vi "counter_polling.vi"() -> ()   [LabVIEW 2018]
panel:
  in  "Button":bool
  in  "stop":bool
  out "Count":u32
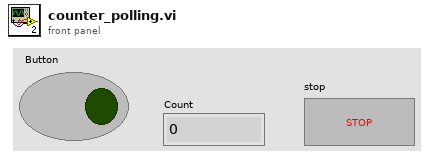
[diagram p1: front panel]
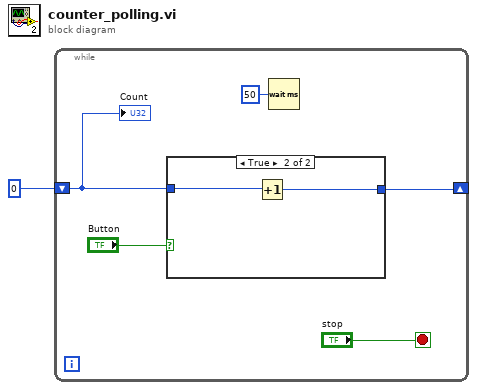
[diagram p0: block diagram]
diagram:
  n1 = while {
    shift-right: [w2] -> _
    shift-left: u32 0 ("milliseconds to wait") -> [w3]
    stop <- "stop" stop-if-true
    n2 = case shown="True" "Button" {
      tunnel: w3 -> [w7 w9]
      tunnel: [w7 w8] -> w2
      frame False {
      }
      frame True {
        n3 = Increment(x=w9) -> (x+1=w8:u32)
      }
    }
    n4 = Wait (ms)(milliseconds to wait=u32 50) -> ()  [unwired: 1 out]
    "Count" <- w3
  }
